vi "Parse Bitfile Version.vi"(11 "EST version string":string) -> (2 "valid":bool, 3 "EST version enum":T1)   [LabVIEW 2013, in "Engine Simulation Session.lvclass"]
uses:
  Engine Simulation Session.lvclass
  Bitfile Major Version.ctl
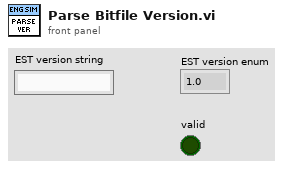
[diagram p1: front panel]
types:
  T1 = typedef "Engine Simulation Session.lvclass/Bitfile Major Version.ctl" = enum16{"1.0", "1.1", "1.2", "1.3"}
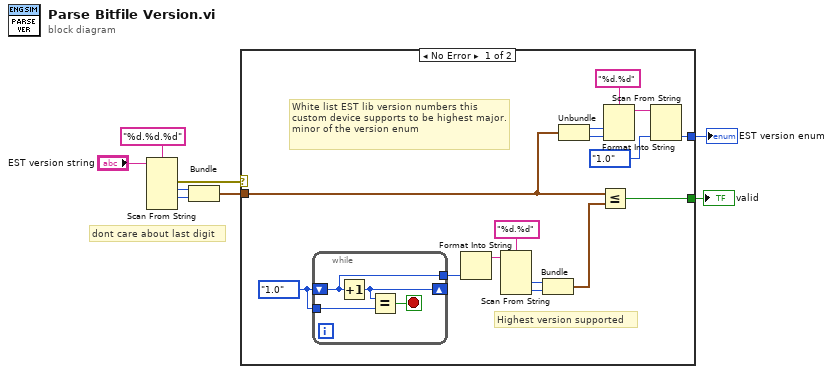
[diagram p0: block diagram]
diagram:
  # "dont care about last digit"
  n1 = Scan From String(format string="%d.%d.%d", input string="EST version string") -> (error out=w4:errorcluster, output 1=w7:i32, output 2=w8:i32)  [unwired: 6 in, 2 out]
  n2 = Bundle(w7, w8) -> (w3:cluster{i32, i32})  [unwired: 1 in]
  n3 = case shown="No Error" w4 {
    tunnel: w3 -> [w15 _]
    tunnel: [w12 _] -> w2
    tunnel: [w9 _] -> w1
    frame No Error {
      w18 = Bitfile_Major_Version."1.0" ("Version")
      # "White list EST lib version numbers this custom device supports to be highest major.minor of the version enum"
      # "Highest version supported"
      n4 = while {
        shift-right: [w25] -> _
        shift-left: w18 -> [w27]
        tunnel: [w27] -> w19
        tunnel: w18 -> [w24]
        stop <- w26 stop-if-true
        n5 = Increment(x=w27) -> (x+1=w25:T1)
        n6 = Equal?(x=w25, y=w24) -> (x = y?=w26:bool)
      }
      n7 = Format Into String(w19) -> (resulting string=w23:string)  [unwired: 3 in, 1 out]
      n8 = Scan From String(format string="%d.%d", input string=w23) -> (output 1=w21:i32, output 2=w20:i32)  [unwired: 4 in, 3 out]
      n9 = Bundle(w21, w20) -> (w17:cluster{i32, i32})  [unwired: 1 in]
      n10 = Unbundle(w15) -> (w14:i32, w13:i32)
      n11 = Less Or Equal?(x=w15, y=w17) -> (x <= y?=w12:bool)
      n12 = Format Into String(format string="%d.%d", w14, w13) -> (resulting string=w11:string)  [unwired: 2 in, 1 out]
      n13 = Scan From String(input string=w11, default 1=Bitfile_Major_Version."1.0" ("Version")) -> (output 1=w9:T1)  [unwired: 3 in, 3 out]
    }
    frame Error {
    }
  }
  "EST version enum" <- w1
  "valid" <- w2
